vi "Mentés.vi"(8 "error in":errorcluster, 11 "Felhasználói adatok in":string[][](array[string])) -> (0 "error out":errorcluster)   [LabVIEW 2014]
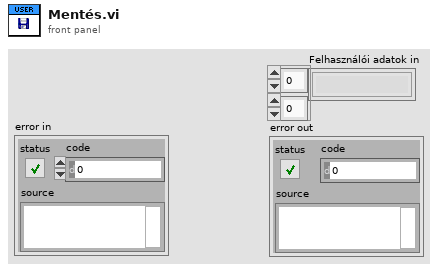
[diagram p1: front panel]
types:
  T1 = cluster{"Felhasználói adatok in[0]":string, "Felhasználói adatok in[1]":string, "Felhasználói adatok in[2]":string}
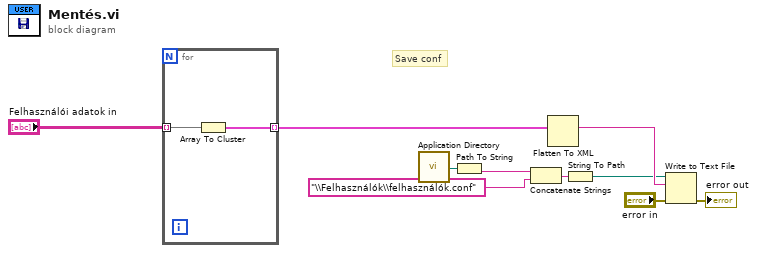
[diagram p0: block diagram]
diagram:
  # "Save conf"
  n1 = for {
    tunnel: "Felhasználói adatok in" -> [w12] mode=indexing
    tunnel: [w11] -> w3 mode=indexing
    n2 = Array To Cluster(array=w12) -> (cluster=w11:T1)
  }
  n3 = call <vilib>:"Application Directory.vi"() -> ("Application Directory"=w9:path)
  n4 = Path To String(path=w9) -> (string=w7:string)
  n5 = Concatenate Strings(w7, "\\Felhasználók\\felhasználók.conf" ("prompt (Choose or enter file path)")) -> (w8:string)
  n6 = Flatten To XML(anything=w3) -> (xml string=w10:string)
  n7 = String To Path(string=w8) -> (path=w5:path)
  n8 = Write to Text File(file (use dialog)=w5, text=w10, error in="error in") -> (error out=→"error out":errorcluster)  [unwired: 1 in, 2 out]
